vi "SPADQ_DisarmArmTrigger.vi"(8 "error in (no error)":errorcluster, 9 "adq_num":i32, 10 "adq_cu_ptr in":refnum<k24>, 11 "ADQAPI Ref":refnum<k24>) -> (0 "error out":errorcluster, 3 "ADQAPI Ref (out)":refnum<k24>)   [LabVIEW 2022 SP3]
doc: "_____AlazarTech, Scope_____\n\nSet the Trigger delay"
uses:
  C:/Windows/System32/ADQAPI_dotNet_helper.dll
panel:
  out "return":i32
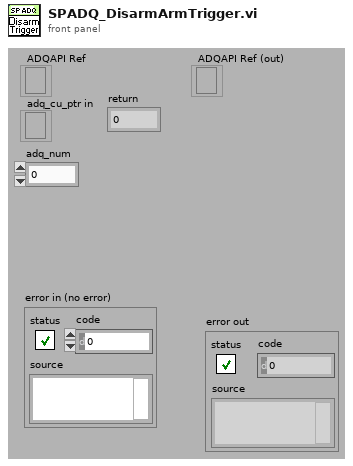
[diagram p1: front panel]
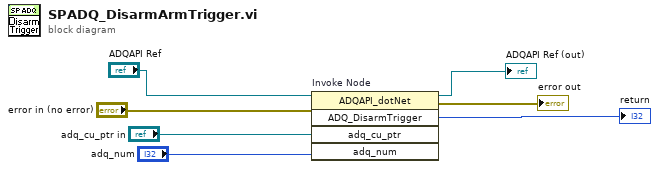
[diagram p0: block diagram]
diagram:
  n1 = invoke on="Invoke Node" class="ADQAPI_dotNet" method="ADQ_DisarmTrigger"(reference="ADQAPI Ref", error in="error in (no error)", "adq_cu_ptr"="adq_cu_ptr in", "adq_num"="adq_num") -> (reference out=→"ADQAPI Ref (out)":refnum<k24>, error out=→"error out":errorcluster, "ADQ_DisarmTrigger"=→"return":i32)  [unwired: 1 in, 2 out]
